vi "process_error_handler.vi"() -> ()   [LabVIEW 2010]
uses:
  typedefs/main_state_enum.ctl
  globals/exit.vi
panel:
  out "error out":errorcluster
  in  "error in (no error)":errorcluster
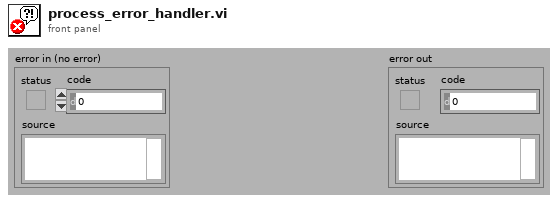
[diagram p1: front panel]
types:
  T1 = typedef "main_state_enum.ctl" = enum16{"Init", "Empty", "ParamsChanged", "Start", "Stop", "Abort", "Acquisition finished", "SetShutter", "Reset", "Error", "Quit"}
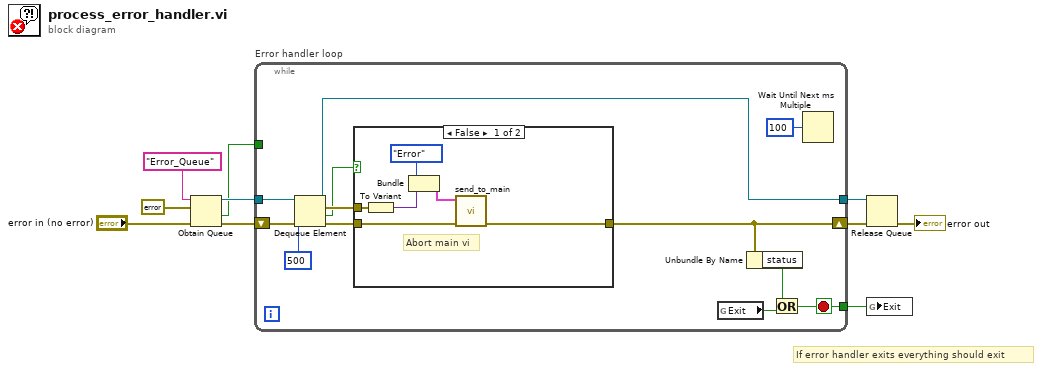
[diagram p0: block diagram]
diagram:
  # "If error handler exits everything should exit"
  n1 = Obtain Queue(name (unnamed)="Error_Queue", element data type=errorcluster {"status"=FALSE, "code"=0, "source"=""} ("error in (no error)"), error in (no error)="error in (no error)") -> (queue out=w7:refnum<queue>, created new?=w1:bool, error out=w8:errorcluster)  [unwired: 2 in]
  n2 = while "Error handler loop" {
    tunnel: w7 -> [w21]
    tunnel: [w19] -> w5
    shift-right: [w18] -> w6
    shift-left: w8 -> [w22]
    tunnel: [w15] -> w2
    tunnel: w1 -> [_]
    stop <- w15 stop-if-true
    n3 = Dequeue Element(queue=w21, timeout in ms (-1)=500, error in (no error)=w22) -> (queue out=w19:refnum<queue>, element=w20:errorcluster, timed out?=w12:bool, error out=w11:errorcluster)
    n4 = case shown="False" w12 {
      tunnel: w20 -> [w26 _]
      tunnel: [w28 w29] -> w18
      tunnel: w11 -> [w27 w29]
      frame False {
        # "Abort main vi"
        n5 = To Variant(anything=w26) -> (Variant=w24:variant)
        n6 = Bundle("Main state"=main_state_enum."Error", "Variant"=w24) -> (w23:cluster{"Main state":T1, "Variant":variant})  [unwired: 1 in]
        n7 = call "send_to_main.vi"("error in (no error)"=w27, "Main state cluster"=w23) -> ("error out"=w28:errorcluster)  [unwired: 9 in]
      }
      frame True {
      }
    }
    n8 = global read "exit.vi" "Exit"() -> (w17:bool)
    n9 = Unbundle By Name(w18) -> ("status"=w16:bool)
    n10 = Or(x=w16, y=w17) -> (x .or. y?=w15:bool)
    n11 = Wait Until Next ms Multiple(millisecond multiple=u32 100) -> ()  [unwired: 1 out]
  }
  n12 = Release Queue(queue=w5, error in (no error)=w6) -> (error out=→"error out":errorcluster)  [unwired: 1 in, 2 out]
  n13 = global write "exit.vi" "Exit"(w2) -> ()
